vi "Disconnect.vi"(8 "Error In":errorcluster, 10 "Description":string="Normal Shutdown", 11 "Session In":refnum<class "Session.lvclass">) -> (0 "Error Out":errorcluster, 3 "Sesssion Out":refnum<class "Session.lvclass">)   [LabVIEW 2021, in "Field_RnD_Services_LIBSSH2_Toolkit.lvlib" / "Session.lvclass"]
doc: "Disconnects a session from a remote SSH server. The user will need to be re-authenticated after the session is disconnected. This is typically called immediate BEFORE destroying the session. This does NOT free the underlying resource within the libssh2 shared library."
uses:
  Session.lvclass
  Session.lvclass/Session.ctl
  Field_RnD_Services_LIBSSH2_Toolkit.lvlib
  SSH/SSH.lvclass
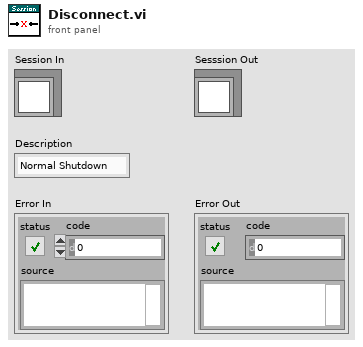
[diagram p1: front panel]
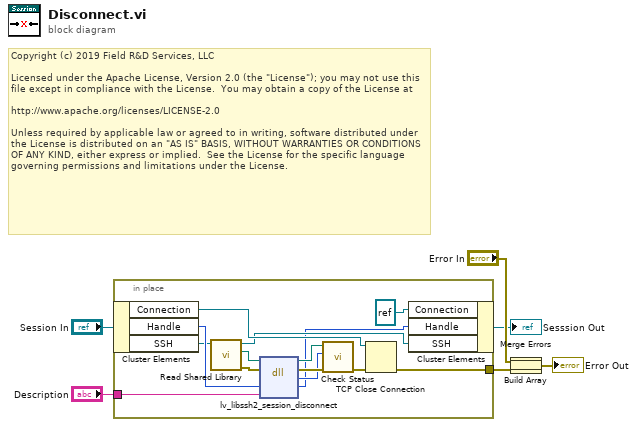
[diagram p0: block diagram]
diagram:
  # "Copyright (c) 2019 Field R&D Services, LLC\n\nLicensed under the Apache License, Version 2.0 (the \"License\"); you may not use this file except in compliance with the License.  You may obtain a copy of the License at\n\nhttp://www.apache.org/licenses/LICENSE-2.0\n\nUnless required by applicable law or agreed to in writing, software distributed under the License is distributed on an \"AS IS\" BASIS, WITHOUT WARRANTIES OR CONDITIONS OF ANY KIND, either express or implied.  See the License for the specific language governing permissions and limitations under the License."
  n1 = in-place {
    in-place-border: "Description" -> [w19]
    in-place-border: [w18] -> w2
    n2 = in-place-cluster #1("Session In") -> ("Connection"=w21:refnum<k5>, "Handle"=w17:u64, "SSH"=w12:refnum<class "SSH.lvclass">)
    n3 = call "Read Shared Library.vi"("SSH In"=w12) -> ("Error Out"=w10:errorcluster, "libssh2lv Shared Library"=w9:path, "SSH Out"=w11:refnum<class "SSH.lvclass">)  [unwired: 8 in]
    n4 = dll-call lib="libssh2lv.*" fn="lv_libssh2_session_disconnect"(path in=w9, error in=w10, "session"=w17, "description"=w19) -> (path out=w15:path, error out=w16:errorcluster, "result"=w13:i32, "session"=w8:u64)  [unwired: 2 in]
    n5 = call "Check Status.vi"("Error In"=w16, "Status"=w13, "libssh2lv Shared Library In"=w15) -> ("Error Out"=w14:errorcluster)  [unwired: 7 in, 1 out]
    n6 = TCP Close Connection(connection ID=w21, error in (no error)=w14) -> (error out=w18:errorcluster)  [unwired: 1 in, 1 out]
    n7 = in-place-cluster #1("Connection"=refnum<k5> refnum, "Handle"=w8, "SSH"=w11) -> (→"Sesssion Out":refnum<class "Session.lvclass">)
  }
  n8 = Build Array("Error In", w2) -> (w1:errorcluster[])
  n9 = Merge Errors(w1) -> (→"Error Out":errorcluster)
